vi "Caller VI_Get Monochrome Image Data.vi"() -> (3 "monochrome":T1)   [LabVIEW 2021]
uses:
  <vilib>/picture/picture.llb/imagedata.ctl
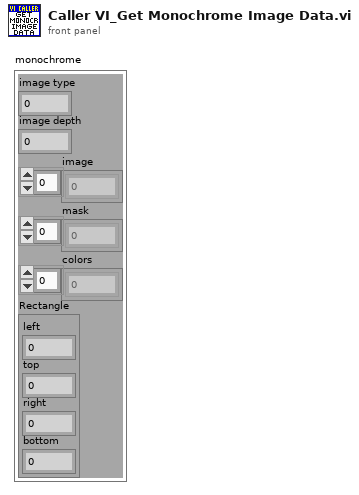
[diagram p1: front panel]
types:
  T1 = typedef "imagedata.ctl" = cluster{"image type":i32, "image depth":i32, "image":u8[], "mask":u8[], "colors":u32[], "Rectangle":cluster{"left":i16, "top":i16, "right":i16, "bottom":i16}}
  T2 = typedef "Who Invoked Icon Editor.ctl" = cluster{"Icon Editor Invoker Type":T3, "App Refnum of Invoker":refnum<vi>, "Qualified Name of Invoker":string, "Path to Invoker":path}
  T3 = typedef "Icon Editor Invoker Type.ctl" = enum32{"Unknown Icon Source", "VI Icon", "Library Icon (any library type)", "Palette icon", "Icon from App Method"}
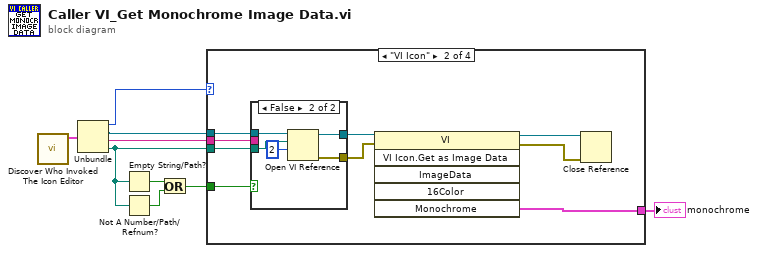
[diagram p0: block diagram]
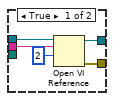
[diagram p3: hidden frame]
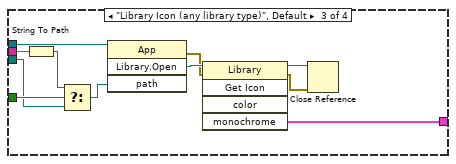
[diagram p4: hidden frame]
diagram:
  n1 = call <resource>:"Discover Who Invoked The Icon Editor.vi"() -> ("Who Invoked The Icon Editor?"=w9:T2)  [unwired: 11 out]
  n2 = Unbundle(w9) -> ("Icon Editor Invoker Type"=w7:T3, "App Refnum of Invoker"=w8:refnum<vi>, "Qualified Name of Invoker"=w3:string, "Path to Invoker"=w2:path)
  n3 = Empty String/Path?(string/path=w2) -> (empty?=w6:bool)
  n4 = Not A Number/Path/Refnum?(number/path/refnum=w2) -> (NaN/Path/Refnum?=w5:bool)
  n5 = Or(x=w6, y=w5) -> (x .or. y?=w4:bool)
  n6 = case shown="\"VI Icon\"" w7 {
    tunnel: w8 -> [_ w16 w37 _]
    tunnel: w3 -> [_ w14 w33 _]
    tunnel: w2 -> [_ w13 w34 _]
    tunnel: w4 -> [_ w15 w35 _]
    tunnel: [_ w10 w29 _] -> w1
    frame "Unknown Icon Source" {
    }
    frame "VI Icon" {
      n7 = case shown="False" w15 {
        tunnel: [w23 w28] -> w18
        tunnel: [w22 w27] -> w17
        tunnel: w16 -> [w21 w26]
        tunnel: w14 -> [w20 _]
        tunnel: w13 -> [_ w25]
        frame True {
          n8 = Open VI Reference(application reference (local)=w21, vi path=w20, options=2) -> (vi reference=w23:refnum<vi>, error out=w22:errorcluster)  [unwired: 1 in, 2 out]
        }
        frame False {
          n9 = Open VI Reference(application reference (local)=w26, vi path=w25, options=2) -> (vi reference=w28:refnum<vi>, error out=w27:errorcluster)  [unwired: 1 in, 2 out]
        }
      }
      n10 = invoke class="VI" method="VI Icon.Get as Image Data"(reference=w18, error in=w17) -> (reference out=w12:refnum<vi>, error out=w11:errorcluster, "Monochrome"=w10:T1)  [unwired: 4 in, 3 out]
      n11 = Close Reference(reference=w12, error in (no error)=w11) -> ()  [unwired: 1 out]
    }
    frame "Library Icon (any library type)", Default {
      n12 = String To Path(string=w33) -> (path=w32:path)
      n13 = Select(t=w32, s=w35, f=w34) -> (s? t:f=w31:path)
      n14 = invoke class="App" method="Library.Open"(reference=w37, "path"=w31) -> (error out=w36:errorcluster, "Open Library"=w39:refnum<vi>)  [unwired: 2 in, 2 out]
      n15 = invoke class="Library" method="Get Icon"(reference=w39, error in=w36) -> (reference out=w38:refnum<vi>, error out=w30:errorcluster, "monochrome"=w29:T1)  [unwired: 3 in, 2 out]
      n16 = Close Reference(reference=w38, error in (no error)=w30) -> ()  [unwired: 1 out]
    }
    frame "Palette icon" {
    }
  }
  "monochrome" <- w1
